vi "unflattenForceFromXML.vi"   [LabVIEW 2012, in "UnitsAndXML.lvlib"]
doc: "Generates time in the unit specified in <B>forceUnitInXML</B> from the data in <B>xmlString</B>, where the source unit is <B>forceUnitInXML</B>. The VI uses <B>forceForType</B> to select the appropriate polymorphic method."
uses:
  <userlib>/Common/UnitsAndXML/UnitsAndXML.lvlib
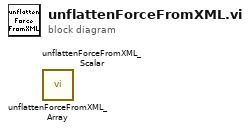
[diagram p0: block diagram]
diagram:
  n1 = call <userlib>:"unflattenForceFromXML_Array.vi"() -> ()  [unwired: 10 in, 2 out]
  n2 = call <userlib>:"unflattenForceFromXML_Scalar.vi"() -> ()  [unwired: 10 in, 2 out]
